vi "save_data_stop.vi"(10 "Avi Refnum":T1, 11 "Data refnum":refnum<file>) -> ()   [LabVIEW 2019]
uses:
  <vilib>/vision/Avi1.llb/AviRefnum.ctl
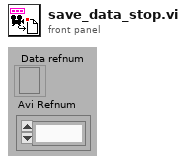
[diagram p1: front panel]
types:
  T1 = typedef "AviRefnum.ctl" = refnum<k1>
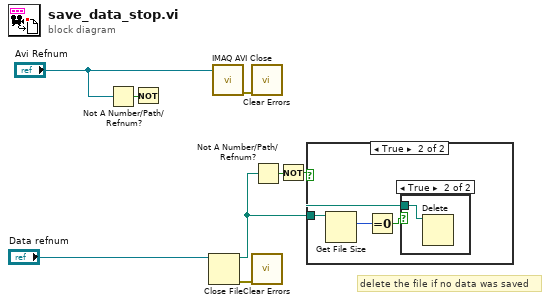
[diagram p0: block diagram]
diagram:
  # "delete the file if no data was saved"
  n1 = Not A Number/Path/Refnum?(number/path/refnum="Avi Refnum") -> (NaN/Path/Refnum?=w7:bool)
  n2 = Not(x=w7) -> ()  [unwired: 1 out]
  n3 = Close File(refnum="Data refnum") -> (path=w2:path, error out=w4:errorcluster)  [unwired: 1 in]
  n4 = call "IMAQ AVI Close"("Avi Refnum"="Avi Refnum") -> ("error out"=w3:errorcluster)  [unwired: 10 in]
  n5 = call <vilib>:"Clear Errors.vi"("error in (no error)"=w3) -> ()  [unwired: 5 in, 2 out]
  n6 = call <vilib>:"Clear Errors.vi"("error in (no error)"=w4) -> ()  [unwired: 5 in, 2 out]
  n7 = Not A Number/Path/Refnum?(number/path/refnum=w2) -> (NaN/Path/Refnum?=w6:bool)
  n8 = Not(x=w6) -> (.not. x?=w1:bool)
  n9 = case shown="True" w1 {
    tunnel: w2 -> [_ w9]
    frame False {
    }
    frame True {
      n10 = Get File Size(file=w9) -> (size (in bytes)=w11:i64)  [unwired: 1 in, 2 out]
      n11 = Equal To 0?(x=w11) -> (x = 0?=w10:bool)
      n12 = case shown="True" w10 {
        tunnel: w9 -> [_ w12]
        frame False {
        }
        frame True {
          n13 = Delete(path (use dialog)=w12) -> ()  [unwired: 4 in, 3 out]
        }
      }
    }
  }
